vi "Control_Rack_Controler.vi"(0 "Times":dbl[](array[numeric]), 1 "Voltages Toroidal (Keep below |10|)":dbl[](array[numeric]), 2 "Voltages Helical (Keep below |10|)":dbl[](array[numeric]), 3 "error out":errorcluster, 4 "Data out 2":T2) -> (5 "error out 2":errorcluster, 6 "Data out":T2)   [LabVIEW 2017]
uses:
  Type_Defs/Data.ctl
  Type_Defs/Diagnostics.ctl
  Type_Defs/Systems.ctl
  <vilib>/DAQmx/write.llb/DAQmx Write (Analog DBL 1Chan 1Samp).vi
  <vilib>/DAQmx/create/channels.llb/DAQmx Create Channel (AO-Voltage-Basic).vi
  <vilib>/DAQmx/miscellaneous.llb/DAQmx Fill In Error Info.vi
  <vilib>/express/express shared/transition.llb/Dynamic To Waveform Array.vi
  <vilib>/express/express signal manip/GetorSetDDTAttributes/Set DDT Attributes/SetT0.vi
  <vilib>/express/express shared/transition.llb/Waveform Array To Dynamic.vi
  <vilib>/express/express signal manip/GetorSetDDTAttributes/Set DDT Attributes/Set DDT Properties.xnode
panel:
  out "Experiment State":T1(ring)
  out "Experiment Purpose":string
  out "Start Time":timestamp
  out "Experiment Number":i32
  out "Operator":string
  out "Running":bool
  out "hel_cur":dynamicdata(graph) caption="Helix Current Feedback"
  out "hel_vol":dynamicdata(graph) caption="Helix Voltage Feedback"
  out "hel_cur_set":dynamicdata(graph) caption="Helix Limited Current Set Point"
  out "torr_cur_set":dynamicdata(graph) caption="Torroidal Limited Current Set Point"
  out "torr_vol":dynamicdata(graph) caption="Torroidal Voltage Feedback"
  out "torr_cur":dynamicdata(graph) caption="Torroidal Current Feedback"
  out "Voltage Toroidal":dbl
  out "Time":dbl
  out "Voltage Helical":dbl
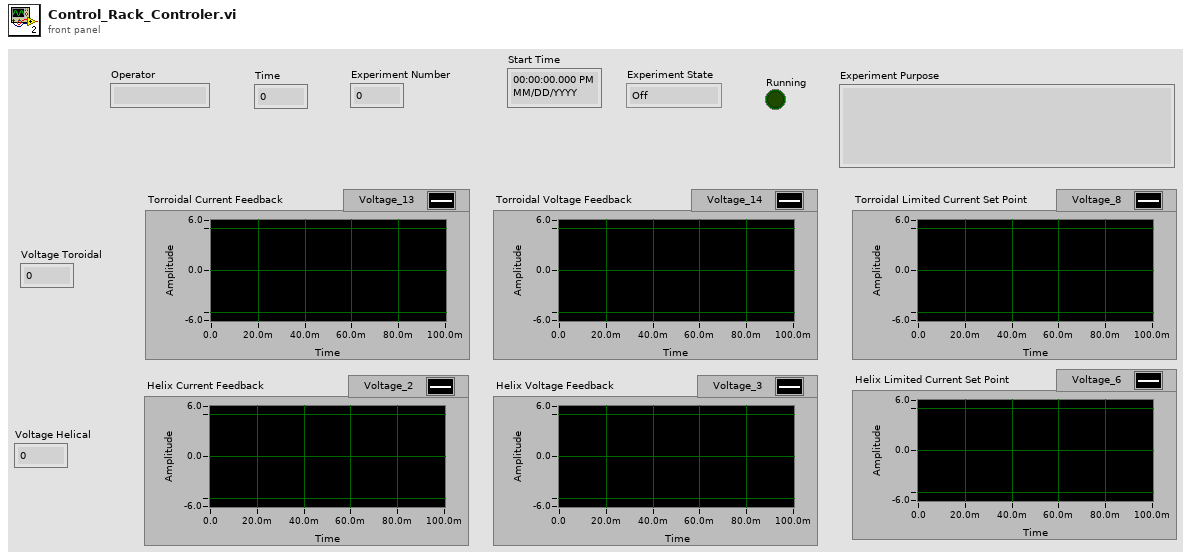
[diagram p1: front panel]
types:
  T1 = enum16{"Off", "Setting Up", "Ready", "In Progress", "Shutting Down"}
  T2 = typedef "Data.ctl" = cluster{"User Name":string, "Experiment Number":i32, "Start Time":timestamp, "Data":dbl[], "Step Number":i32, "Step Instructions":string, "Diagnostics":T3, "Experiment Purpose":string, "Experiment State":enum16{"Off", "Setting Up", "Ready", "In Progress", "Shutting Down"}, "Systems":T4, "Vacuum Pressure":dbl, "Fieldpoints":cluster{"System Boolean Fieldpoints":cluster{"Compressed Air":refnum<k21>, "T-20kV Power Switch":refnum<k21>, "T-Rectifier":refnum<k21>, "Engage Interlock":refnum<k21>, "Ventilator":refnum<k21>, "Magnetron":refnum<k21>, "H-20kV Power Switch":refnum<k21>, "H-Rectifier":refnum<k21>, "Main Water Pump":refnum<k21>, "WEGA Water Pump":refnum<k21>, "Gas Inlet Valves":refnum<k21>}, "Step Fieldpoints":cluster{"Exhaust Ventillator":refnum<k21>, "Compressed Air":refnum<k21>, "Water Pressure":refnum<k21>, "Interlock":refnum<k21>, "Toroidal Power Supply 1":refnum<k21>, "Toroidal Power Supply 2":refnum<k21>, "Toroidal Rectifier":refnum<k21>, "Helical Power Supply":refnum<k21>, "Helical Rectifier":refnum<k21>, "6kW Magnetron Standby":refnum<k21>, "20kW Magnetron Standby":refnum<k21>}}, "Pressure History":cluster{"Seconds into Experiment":i32[], "Pressure Data":dbl[]}, "Time Computer Control":dbl[], "Toroidal Voltage Computer Control":dbl[], "Helical Voltage Computer Control":dbl[], "Toroidal Current":dbl[], "Toroidal Voltage":dbl[], "Toroidal Current Set Point":dbl[], "Helical Current Set Point":dbl[], "Helical Voltage":dbl[], "Helical Current":dbl[], "Experiment Folder":path, "Run Another Shot?":bool}
  T3 = typedef "Diagnostics.ctl" = cluster{"Langmuir Probe":bool, "Rogowski 1":bool, "Rogowski 2":bool, "Rogowski 3":bool, "B-dot 1":bool, "B-dot 2":bool}
  T4 = typedef "Systems.ctl" = cluster{"Compressed Air":bool, "T-20kV Power Switch":bool, "T-Rectifier":bool, "Engage Interlock":bool, "Ventilator":bool, "Magnetron":bool, "H-20kV Power Switch":bool, "H-Rectifier":bool, "Main Water Pump":bool, "WEGA Water Pump":bool, "Gas Inlet Valves":bool}
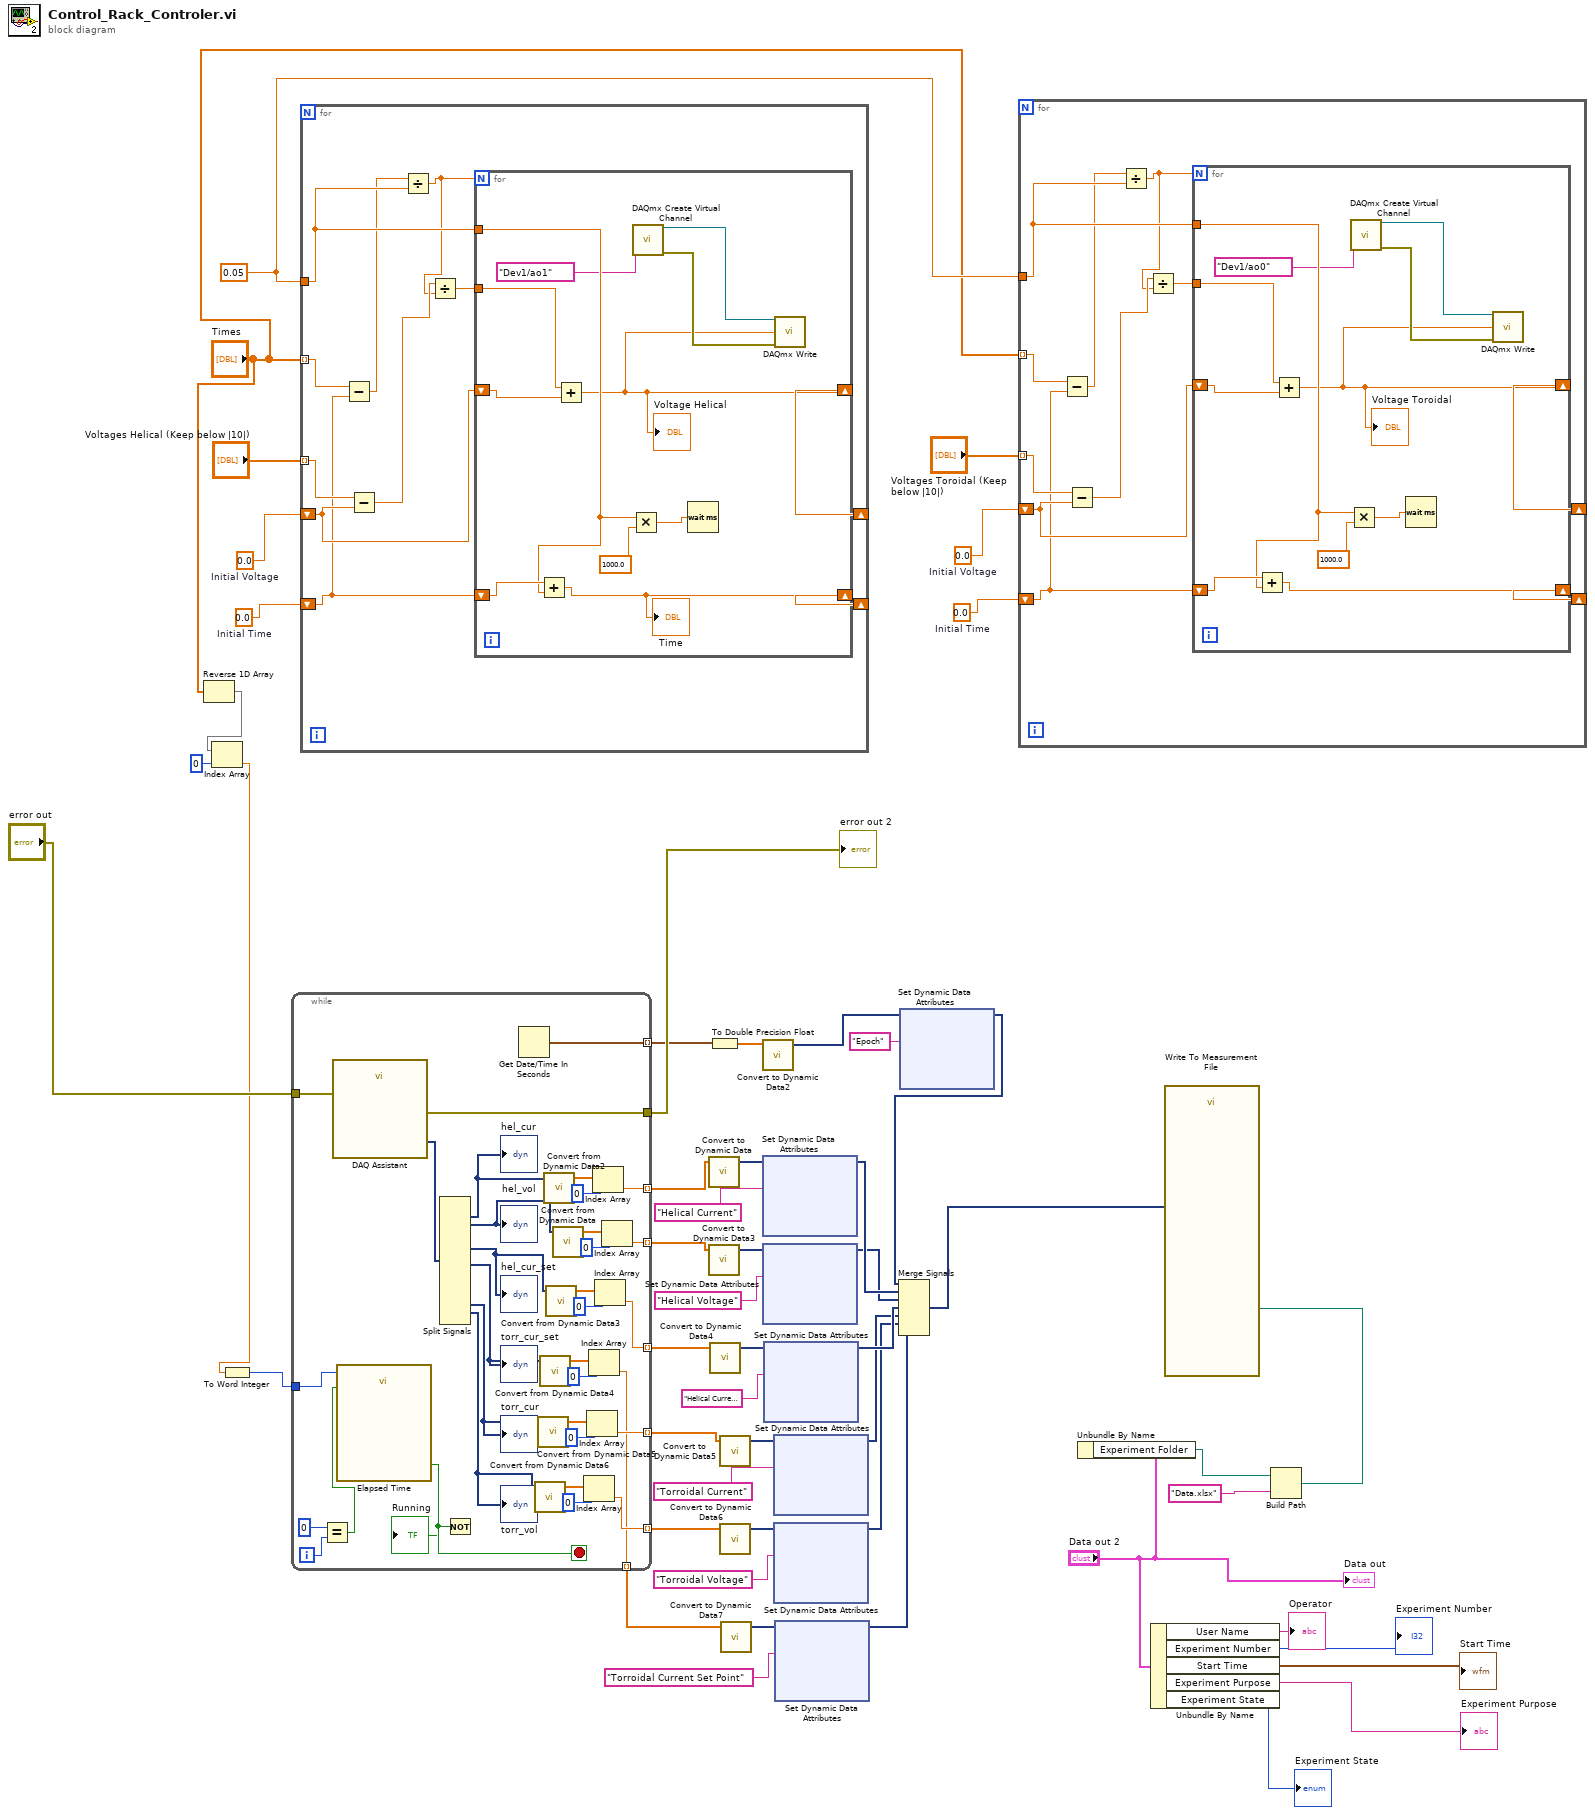
[diagram p0: block diagram]
diagram:
  w47 = 0.05 ("Timestep (in seconds, keep above 1/20s)")
  w50 = 0.0  # Initial Time
  w49 = 0.0  # Initial Voltage
  w51 = 0.0  # Initial Time
  w52 = 0.0  # Initial Voltage
  n1 = Reverse 1D Array(array="Times") -> (reversed array=w45:dbl[])
  n2 = Index Array(array=w45, index=0) -> (element=w41:dbl)
  n3 = To Word Integer(number=w41) -> (16bit integer=w40:i16)
  n4 = while {
    tunnel: "error out" -> [w86]
    tunnel: [w85] -> w42
    tunnel: w40 -> [w84]
    tunnel: [w80] -> w35 mode=indexing
    tunnel: [w79] -> w33 mode=indexing
    tunnel: [w63] -> w11 mode=indexing
    tunnel: [w62] -> w10 mode=indexing
    tunnel: [w61] -> w9 mode=indexing
    tunnel: [w60] -> w8 mode=indexing
    tunnel: [w59] -> w7 mode=indexing
    i -> [w58]
    stop <- w55 stop-if-true
    n5 = Equal?(x=0, y=w58) -> (x = y?=w56:bool)
    n6 = call "DAQ Assistant"("error in"=w86) -> ("data"=w87:dynamicdata, "error out"=w85:errorcluster)  [unwired: 16 in, 1 out]
    n7 = call "Elapsed Time"("Time Target (s)"=w84, "Reset"=w56) -> ("Time has Elapsed"=w55:bool)  [unwired: 10 in, 7 out]
    n8 = Split Signals(w87) -> (w83:dynamicdata, w68:dynamicdata, w67:dynamicdata, w66:dynamicdata, w65:dynamicdata, w64:dynamicdata)  [unwired: 16 in, 10 out]
    "hel_cur" <- w83
    "hel_vol" <- w68
    "hel_cur_set" <- w67
    "torr_cur_set" <- w66
    "torr_vol" <- w64
    "torr_cur" <- w65
    n9 = Not(x=w55) -> (.not. x?=→"Running":bool)
    n10 = Get Date/Time In Seconds() -> (seconds since 1Jan1904=w79:timestamp)
    n11 = call "Convert from Dynamic Data6"("Dynamic Data Type"=w64) -> ("Array"=w70:dbl[])  [unwired: 3 in]
    n12 = call "Convert from Dynamic Data5"("Dynamic Data Type"=w65) -> ("Array"=w72:dbl[])  [unwired: 3 in]
    n13 = call "Convert from Dynamic Data4"("Dynamic Data Type"=w66) -> ("Array"=w74:dbl[])  [unwired: 3 in]
    n14 = call "Convert from Dynamic Data2"("Dynamic Data Type"=w83) -> ("Array"=w82:dbl[])  [unwired: 3 in]
    n15 = call "Convert from Dynamic Data3"("Dynamic Data Type"=w67) -> ("Array"=w76:dbl[])  [unwired: 3 in]
    n16 = call "Convert from Dynamic Data"("Dynamic Data Type"=w68) -> ("Array"=w78:dbl[])  [unwired: 3 in]
    n17 = Index Array(array=w70, index=0) -> (element=w60:dbl)
    n18 = Index Array(array=w72, index=0) -> (element=w61:dbl)
    n19 = Index Array(array=w74, index=0) -> (element=w59:dbl)
    n20 = Index Array(array=w82, index=0) -> (element=w80:dbl)
    n21 = Index Array(array=w76, index=0) -> (element=w62:dbl)
    n22 = Index Array(array=w78, index=0) -> (element=w63:dbl)
  }
  "error out 2" <- w42
  n23 = for {
    tunnel: "Voltages Helical (Keep below |10|)" -> [w98] mode=indexing
    tunnel: "Times" -> [w91] mode=indexing
    tunnel: w47 -> [w93]
    shift-right: [w94] -> _
    shift-left: w52 -> [w97]
    shift-right: [w92] -> _
    shift-left: w51 -> [w90]
    n24 = Subtract(x=w91, y=w90) -> (x-y=w89:dbl)
    n25 = Subtract(x=w98, y=w97) -> (x-y=w96:dbl)
    n26 = Divide(x=w89, y=w93) -> (x/y=w88:dbl)
    n27 = Divide(x=w96, y=w88) -> (x/y=w95:dbl)
    n28 = for {
      N: w88 -> [_]
      shift-right: [w99] -> w94
      shift-left: w97 -> [w109]
      tunnel: w95 -> [w108]
      tunnel: w93 -> [w105]
      shift-right: [w103] -> w92
      shift-left: w90 -> [w107]
      n29 = Add(x=w107, y=w105) -> (x+y=w103:dbl)
      "Time" <- w103
      n30 = Add(x=w108, y=w109) -> (x+y=w99:dbl)
      "Voltage Helical" <- w99
      n31 = Multiply(x=w105, y=1000.0) -> (x*y=w106:dbl)
      n32 = call-poly <vilib>:"DAQmx Create Virtual Channel.vi"("physical channels"=tag "Dev1/ao1" ("write channel (torr = ao0, hel = ao1)")) -> ("task out"=w100:refnum<k21>, "error out"=w101:errorcluster)  [unwired: 13 in]
      n33 = Wait (ms)(milliseconds to wait=w106) -> ()  [unwired: 1 out]
      n34 = call-poly <vilib>:"DAQmx Write.vi"("task/channels in"=w100, "data"=w99, "error in"=w101) -> ()  [unwired: 10 in, 3 out]
    }
  }
  n35 = call "Convert to Dynamic Data"("Array"=w35) -> ("Dynamic Data Type"=w36:dynamicdata)  [unwired: 3 in]
  n36 = call "Convert to Dynamic Data3"("Array"=w11) -> ("Dynamic Data Type"=w26:dynamicdata)  [unwired: 3 in]
  n37 = To Double Precision Float(number=w33) -> (double precision float=w32:dbl[])
  n38 = call "Convert to Dynamic Data4"("Array"=w10) -> ("Dynamic Data Type"=w25:dynamicdata)  [unwired: 3 in]
  n39 = call "Convert to Dynamic Data5"("Array"=w9) -> ("Dynamic Data Type"=w24:dynamicdata)  [unwired: 3 in]
  n40 = call "Convert to Dynamic Data6"("Array"=w8) -> ("Dynamic Data Type"=w22:dynamicdata)  [unwired: 3 in]
  n41 = call "Convert to Dynamic Data7"("Array"=w7) -> ("Dynamic Data Type"=w21:dynamicdata)  [unwired: 3 in]
  n42 = call "Convert to Dynamic Data2"("Array"=w32) -> ("Dynamic Data Type"=w31:dynamicdata)  [unwired: 3 in]
  n43 = xnode "Set Dynamic Data Attributes"("Signals In"=w36, "Signal Name"="Helical Current") -> ("Signals Out"=w29:dynamicdata)  [unwired: 2 in, 1 out]
  n44 = xnode "Set Dynamic Data Attributes"("Signals In"=w26, "Signal Name"="Helical Voltage") -> ("Signals Out"=w20:dynamicdata)  [unwired: 2 in, 1 out]
  n45 = xnode "Set Dynamic Data Attributes"("Signals In"=w25, "Signal Name"="Helical Current Set Point") -> ("Signals Out"=w19:dynamicdata)  [unwired: 2 in, 1 out]
  n46 = xnode "Set Dynamic Data Attributes"("Signals In"=w24, "Signal Name"="Torroidal Current") -> ("Signals Out"=w18:dynamicdata)  [unwired: 2 in, 1 out]
  n47 = xnode "Set Dynamic Data Attributes"("Signals In"=w22, "Signal Name"="Torroidal Voltage") -> ("Signals Out"=w17:dynamicdata)  [unwired: 2 in, 1 out]
  n48 = xnode "Set Dynamic Data Attributes"("Signals In"=w21, "Signal Name"="Torroidal Current Set Point") -> ("Signals Out"=w16:dynamicdata)  [unwired: 2 in, 1 out]
  n49 = xnode "Set Dynamic Data Attributes"("Signals In"=w31, "Signal Name"="Epoch") -> ("Signals Out"=w28:dynamicdata)  [unwired: 2 in, 1 out]
  n50 = Merge Signals(w28, w29, w20, w19, w18, w17, w16) -> (w27:dynamicdata)
  n51 = for {
    tunnel: "Voltages Toroidal (Keep below |10|)" -> [w120] mode=indexing
    tunnel: "Times" -> [w113] mode=indexing
    tunnel: w47 -> [w115]
    shift-right: [w116] -> _
    shift-left: w49 -> [w119]
    shift-right: [w114] -> _
    shift-left: w50 -> [w112]
    n52 = Subtract(x=w113, y=w112) -> (x-y=w111:dbl)
    n53 = Subtract(x=w120, y=w119) -> (x-y=w118:dbl)
    n54 = Divide(x=w111, y=w115) -> (x/y=w110:dbl)
    n55 = Divide(x=w118, y=w110) -> (x/y=w117:dbl)
    n56 = for {
      N: w110 -> [_]
      shift-right: [w121] -> w116
      shift-left: w119 -> [w131]
      tunnel: w117 -> [w130]
      tunnel: w115 -> [w127]
      shift-right: [w125] -> w114
      shift-left: w112 -> [w129]
      n57 = Add(x=w129, y=w127) -> (x+y=w125:dbl)
      n58 = Add(x=w130, y=w131) -> (x+y=w121:dbl)
      "Voltage Toroidal" <- w121
      n59 = Multiply(x=w127, y=1000.0) -> (x*y=w128:dbl)
      n60 = call-poly <vilib>:"DAQmx Create Virtual Channel.vi"("physical channels"=tag "Dev1/ao0" ("write channel (torr = ao0, hel = ao1) 2")) -> ("task out"=w122:refnum<k21>, "error out"=w123:errorcluster)  [unwired: 13 in]
      n61 = Wait (ms)(milliseconds to wait=w128) -> ()  [unwired: 1 out]
      n62 = call-poly <vilib>:"DAQmx Write.vi"("task/channels in"=w122, "data"=w121, "error in"=w123) -> ()  [unwired: 10 in, 3 out]
    }
  }
  n63 = Unbundle By Name("Data out 2") -> ("Experiment Folder"=w38:path)
  n64 = Unbundle By Name("Data out 2") -> ("User Name"=→"Operator":string, "Experiment Number"=→"Experiment Number":i32, "Start Time"=→"Start Time":timestamp, "Experiment Purpose"=→"Experiment Purpose":string, "Experiment State"=→"Experiment State":T1)
  n65 = Build Path(base path=w38, name or relative path="Data.xlsx") -> (appended path=w39:path)
  n66 = call "Write To Measurement File"("Signals"=w27, "Filename"=w39) -> ()  [unwired: 15 in, 3 out]
  "Data out" <- "Data out 2"
